vi "Format Error Into String.vi"(8 "error in (no error)":errorcluster, 11 "Message Data":variant) -> (0 "error out":errorcluster, 2 "error?":bool, 3 "message":string)   [LabVIEW 2019, in "Personalities Tool.lvlib"]
doc: "This VI formats an incoming error in the Data terminal into a string.\nThis function also clears the error wire."
uses:
  Personalities Tool.lvlib
  <vilib>/Utility/error.llb/DialogType.ctl
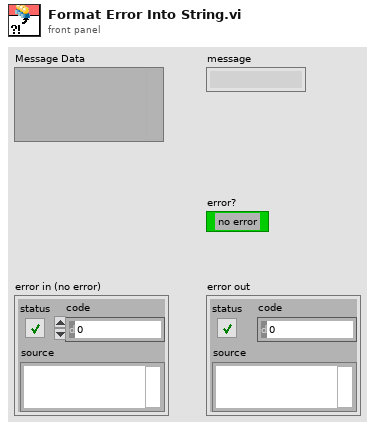
[diagram p1: front panel]
types:
  T1 = typedef "DialogType.ctl" = u16
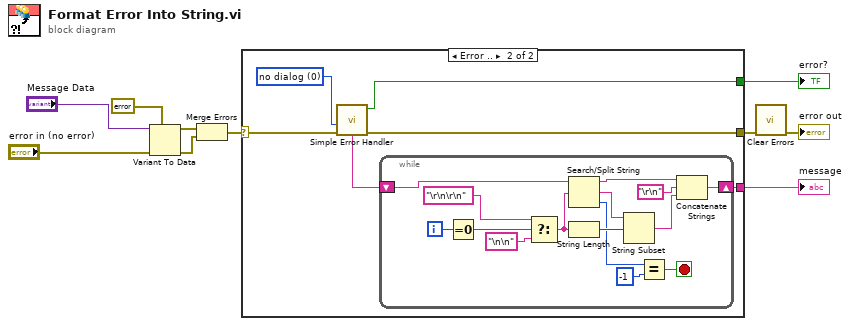
[diagram p0: block diagram]
diagram:
  n1 = Variant To Data(error in="error in (no error)", type=errorcluster {"status"=FALSE, "code"=0, "source"=""} ("error constant"), Variant="Message Data") -> (data=w6:errorcluster, error out=w7:errorcluster)
  n2 = Merge Errors(w6, w7) -> (w9:errorcluster)
  n3 = case shown="Error .." w9 {
    selector: w9 -> [w11 w14]
    tunnel: [_ w17] -> w10
    tunnel: [_ w13] -> w3
    tunnel: [w11 w12] -> w2
    frame No Error {
    }
    frame Error {
      w15 = T1 0 items=["no dialog", "OK message", "continue or stop message", "OK message + warnings", "continue/stop + warnings"] ("type of dialog (OK msg:1)")
      n4 = call <vilib>:"Simple Error Handler.vi"("type of dialog (OK msg:1)"=w15, "error in (no error)"=w14) -> ("error?"=w13:bool, "error out"=w12:errorcluster, "message"=w16:string)  [unwired: 3 in, 2 out]
      n5 = while {
        shift-right: [w28] -> w17
        shift-left: w16 -> [w32]
        i -> [w22]
        stop <- w24 stop-if-true
        n6 = Equal To 0?(x=w22) -> (x = 0?=w21:bool)
        n7 = Select(t="\r\n\r\n", s=w21, f="\n\n") -> (s? t:f=w18:string)
        n8 = Search/Split String(string=w32, search string/char (-)=w18) -> (substring before match=w27:string, match + rest of string=w31:string, offset of match=w25:i32)  [unwired: 1 in]
        n9 = String Length(string=w18) -> (length=w30:i32)
        n10 = String Subset(string=w31, offset (0)=w30) -> (substring=w29:string)  [unwired: 1 in]
        n11 = Equal?(x=w25, y=-1) -> (x = y?=w24:bool)
        n12 = Concatenate Strings(w27, "\r\n", w29) -> (w28:string)
      }
    }
  }
  "message" <- w10
  "error?" <- w3
  n13 = call <vilib>:"Clear Errors.vi"("error in (no error)"=w2) -> ("error out"=→"error out":errorcluster)  [unwired: 5 in, 1 out]
